vi "CSM - Break Down Multiple States String.vi"(10 "States":string) -> (2 "Multiple States":string[](array[string]))   [LabVIEW 2017, in "Communicable State Machine.lvlib"]
doc: "### CSM - Break Down Multiple States String.vi\n\nBreak down a string containing multiple lines of CSM state strings into an array of CSM state strings.\n\n-- <b>Controls</b> --\n- <b>States</b>: String containing multiple lines of CSM state strings\n\n-- <b>Indicators</b> --\n- <b>Multiple States</b>: Array of CSM state strings"
uses:
  Communicable State Machine.lvlib
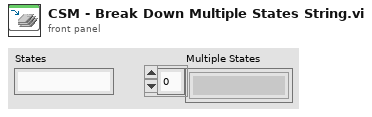
[diagram p1: front panel]
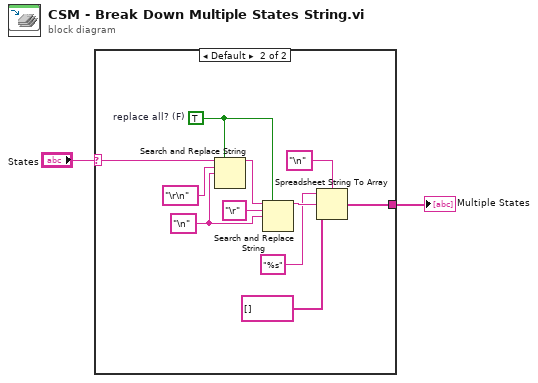
[diagram p0: block diagram]
diagram:
  n1 = case shown="Default" "States" {
    selector: "States" -> [_ w3]
    tunnel: [_ w13] -> w2
    frame "" {
    }
    frame Default {
      w6 = TRUE  # replace all? (F)
      w7 = "\n" ("delimiter (Tab)")
      n2 = Search and Replace String(replace all?=w6, input string=w3, search string="\r\n" ("delimiter (Tab)"), replace string=w7) -> (result string=w8:string)  [unwired: 4 in, 3 out]
      n3 = Search and Replace String(replace all?=w6, input string=w8, search string="\r" ("delimiter (Tab)"), replace string=w7) -> (result string=w11:string)  [unwired: 4 in, 3 out]
      n4 = Spreadsheet String To Array(delimiter (Tab)="\n", format string="%s", spreadsheet string=w11, array type (2D Dbl)=string[] [] ("Array of Strings")) -> (array=w13:string[])
    }
  }
  "Multiple States" <- w2
